vi "Test-DotNet.vi"() -> ()   [LabVIEW 2013, in "EC1000-control.lvlib" / "SM1000-control.lvclass"]
uses:
  SM1000-control.lvclass
  DOTNET-settings.ctl
  Device-identification.ctl
  Fixed-data-type.ctl
  Status-information.ctl
  EC1000_DOTNET/getBroadcastData-status.vi
panel:
  out "serverList iterator":i32
  out "Status information":T1
  out "Job count":i32
  out "Job name list":string
  out "Fixed data":string
  in  "File name wo extension":string="AdminConfig"
  in  "Fixed data type":T2=10 items=["Controller Configuration"=5, "Laser Configuration"=6, "Lens Configuration"=2, "Correction Table"=13, "User Configuration"=15, "Performance Adjustments"=16, "Admin Configuration"=10]
  in  "Device index":i32
  out "piServerCount":i32
  out "Device identifiers":T3[](array[typedef])
  in  "DOTNET settings":T4={"Target IP"="128.178.146.163", "Target broadcast port"=11000, "Target communication port"=12200, "clientID"=-1, "Broadcast IP"="224.168.100.2", "Servercount"=-1, "Device IDs"=[]}
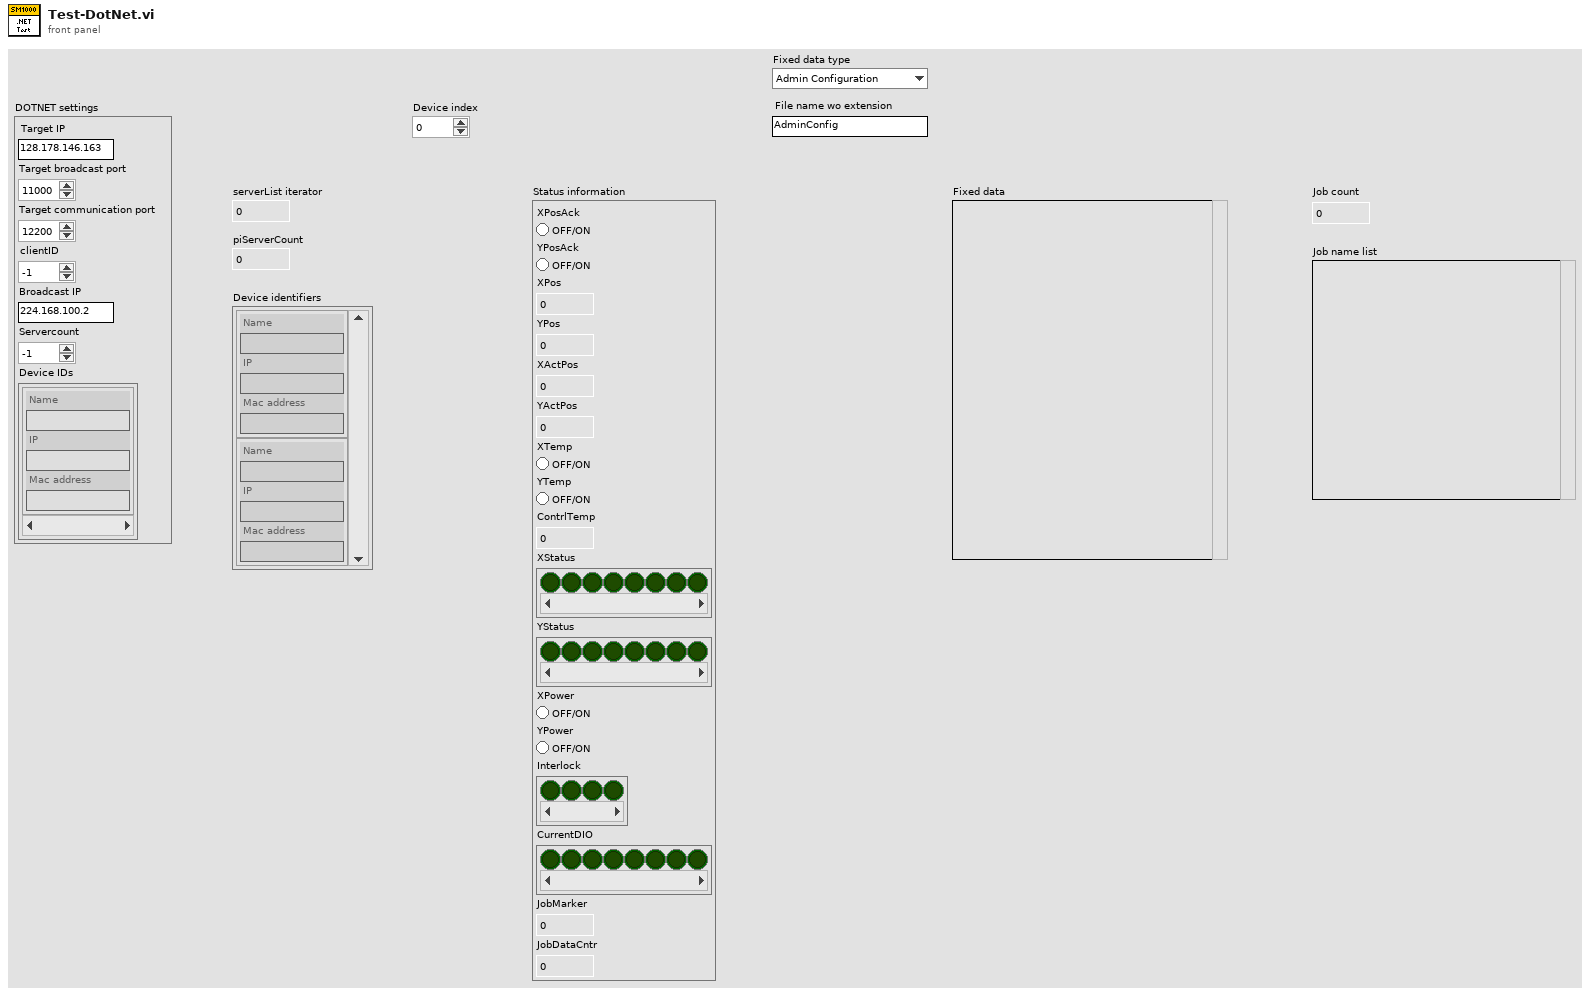
[diagram p1: front panel]
types:
  T1 = typedef "EC1000-control.lvlib/SM1000-control.lvclass/Status-information.ctl" = cluster{"XPosAck":bool, "YPosAck":bool, "XPos":i16, "YPos":i16, "XActPos":i16, "YActPos":i16, "XTemp":bool, "YTemp":bool, "ContrlTemp":i16, "XStatus":bool[], "YStatus":bool[], "XPower":bool, "YPower":bool, "Interlock":bool[], "CurrentDIO":bool[], "JobMarker":u16, "JobDataCntr":u32}
  T2 = typedef "EC1000-control.lvlib/SM1000-control.lvclass/Fixed-data-type.ctl" = i32
  T3 = typedef "EC1000-control.lvlib/SM1000-control.lvclass/Device-identification.ctl" = cluster{"Name":string, "IP":string, "Mac address":string}
  T4 = typedef "EC1000-control.lvlib/SM1000-control.lvclass/DOTNET-settings.ctl" = cluster{"Target IP":string, "Target broadcast port":i32, "Target communication port":i32, "clientID":i32, "Broadcast IP":string, "Servercount":i32, "Device IDs":T3[]}
  T5 = typedef "EC1000-control.lvlib/SM1000-control.lvclass/Object-reference.ctl" = refnum<data-value>
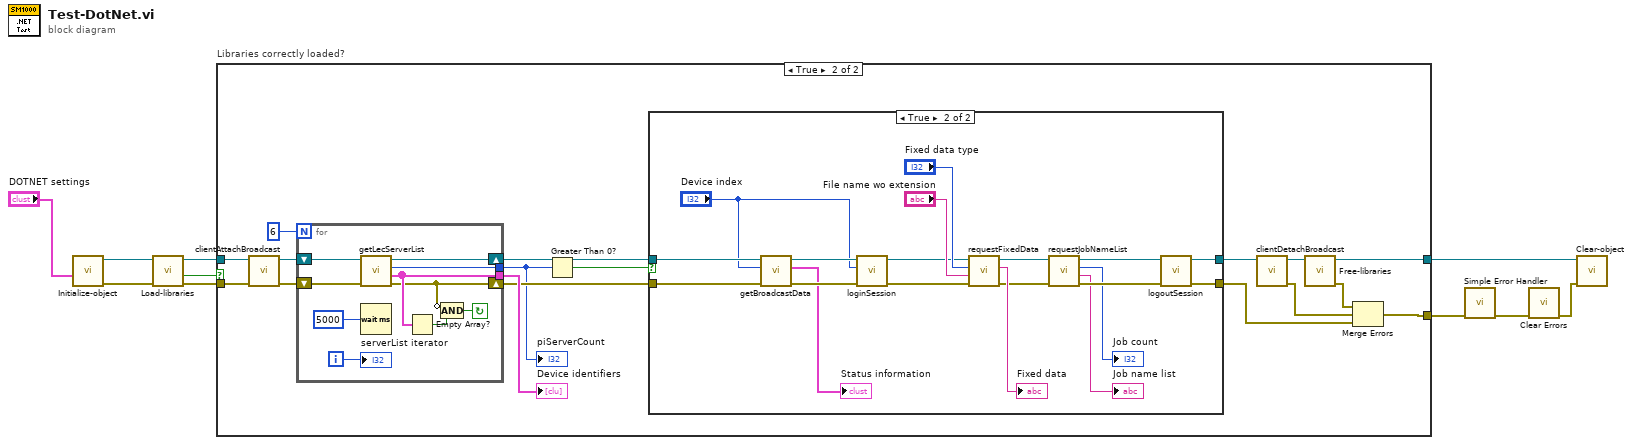
[diagram p0: block diagram]
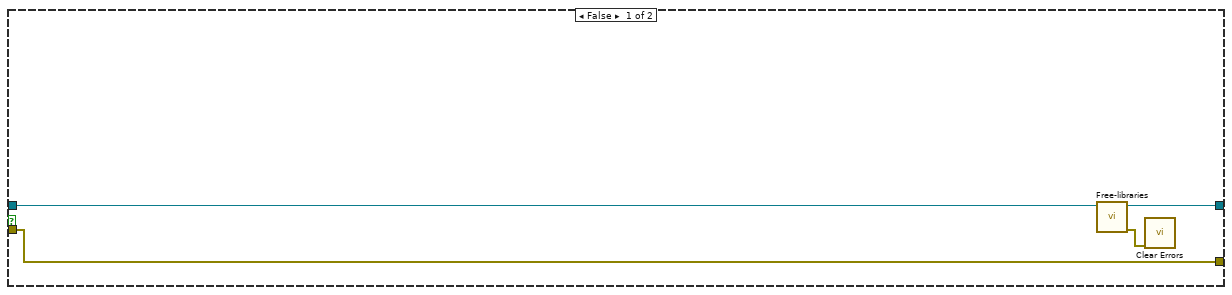
[diagram p2: hidden frame]
diagram:
  n1 = call "Initialize-object.vi"("DOTNET settings"="DOTNET settings") -> ("error out"=w8:errorcluster, "SM1000-control out"=w9:T5)  [unwired: 9 in]
  n2 = call "Load-libraries.vi"("error in (no error)"=w8, "SM1000-control in"=w9) -> ("error out"=w5:errorcluster, "Loaded?"=w7:bool, "SM1000-control out"=w6:T5)  [unwired: 7 in]
  n3 = case "Libraries correctly loaded?" shown="True" w7 {
    tunnel: w6 -> [w13 w28]
    tunnel: w5 -> [w14 w27]
    tunnel: [w14 w30] -> w3
    tunnel: [w12 w29] -> w1
    frame False {
      n4 = call "Free-libraries.vi"("SM1000-control in"=w13) -> ("error out"=w11:errorcluster, "SM1000-control out"=w12:T5)  [unwired: 8 in, 1 out]
      n5 = call <vilib>:"Clear Errors.vi"("error in (no error)"=w11) -> ()  [unwired: 6 in, 1 out]
    }
    frame True {
      n6 = call "clientAttachBroadcast.vi"("error in (no error)"=w27, "SM1000-control in"=w28) -> ("error out"=w23:errorcluster, "SM1000-control out"=w24:T5)  [unwired: 7 in, 1 out]
      n7 = for {
        N: 6 -> [_]
        tunnel: [w57] -> w22
        tunnel: [w60] -> w16
        shift-right: [w59] -> w18
        shift-left: w24 -> [w62]
        shift-right: [w54] -> w17
        shift-left: w23 -> [w61]
        i -> [w56]
        stop <- w53 continue-if-true
        n8 = call "getLecServerList.vi"("error in (no error)"=w61, "SM1000-control in"=w62) -> ("error out"=w54:errorcluster, "Device identifiers"=w57:T3[], "piServerCount"=w60:i32, "SM1000-control out"=w59:T5)  [unwired: 6 in]
        n9 = Wait (ms)(milliseconds to wait=u32 5000) -> ()  [unwired: 1 out]
        n10 = Empty Array?(array=w57) -> (empty?=w55:bool)
        n11 = Compound Arithmetic op=AND(invert w54, w55) -> (w53:bool)
        "serverList iterator" <- w56
      }
      "Device identifiers" <- w22
      "piServerCount" <- w16
      n12 = Greater Than 0?(x=w16) -> (x > 0?=w15:bool)
      n13 = case shown="True" w15 {
        tunnel: [w32 w52] -> w20
        tunnel: [w33 w51] -> w19
        tunnel: w18 -> [w33 w39]
        tunnel: w17 -> [w32 w38]
        frame False {
        }
        frame True {
          n14 = call-poly "getBroadcastData.vi"("error in (no error)"=w38, "Device index"="Device index", "SM1000-control in"=w39) -> ("error out"=w36:errorcluster, "Status information"=→"Status information":T1, "SM1000-control out"=w37:T5)  [unwired: 6 in]
          n15 = call "loginSession.vi"("error in (no error)"=w36, "Device index"="Device index", "SM1000-control in"=w37) -> ("error out"=w47:errorcluster, "SM1000-control out"=w48:T5)  [unwired: 7 in]
          n16 = call "requestFixedData.vi"("error in (no error)"=w47, "File name wo extension"="File name wo extension", "Fixed data type"="Fixed data type", "SM1000-control in"=w48) -> ("error out"=w44:errorcluster, "File contents"=→"Fixed data":string, "SM1000-control out"=w45:T5)  [unwired: 5 in]
          n17 = call "requestJobNameList.vi"("error in (no error)"=w44, "SM1000-control in"=w45) -> ("error out"=w42:errorcluster, "Job name list"=→"Job name list":string, "Job count"=→"Job count":i32, "SM1000-control out"=w43:T5)  [unwired: 6 in]
          n18 = call "logoutSession.vi"("error in (no error)"=w42, "SM1000-control in"=w43) -> ("error out"=w52:errorcluster, "SM1000-control out"=w51:T5)  [unwired: 8 in]
        }
      }
      n19 = call "clientDetachBroadcast.vi"("SM1000-control in"=w19) -> ("error out"=w25:errorcluster, "SM1000-control out"=w26:T5)  [unwired: 9 in]
      n20 = call "Free-libraries.vi"("SM1000-control in"=w26) -> ("error out"=w31:errorcluster, "SM1000-control out"=w29:T5)  [unwired: 8 in, 1 out]
      n21 = Merge Errors(w31, w25, w20) -> (w30:errorcluster)
    }
  }
  n22 = call <vilib>:"Simple Error Handler.vi"("error in (no error)"=w3) -> ("error out"=w4:errorcluster)  [unwired: 4 in, 4 out]
  n23 = call <vilib>:"Clear Errors.vi"("error in (no error)"=w4) -> ("error out"=w2:errorcluster)  [unwired: 6 in]
  n24 = call "Clear-object.vi"("error in (no error)"=w2, "SM1000-control"=w1) -> ()  [unwired: 8 in, 2 out]
